vi "Util_Trajectory_WriteFile_Pathweaver.vi"(6 "Trajectory Is Relative":bool, 8 "UtilityWayPoints":T6[](array[typedef]) {"ANGLE" format="%13.3f"; "Y" format="%13.3f"; "X" format="%13.3f"}, 9 "TRAJECTORY":T1 {"States"."POSE"."ROTATION"."SIN" format="%13.4f"; "States"."POSE"."ROTATION"."COS" format="%13.4f"; "States"."POSE"."ROTATION"."VALUE" format="%13.4f"; "States"."POSE"."TRANSLATION"."Y" format="%14.3f"; "States"."POSE"."TRANSLATION"."X" format="%14.3f"; "TotalTImeSecs" format="%20.3f"}, 10 "Comment":string, 11 "Trajectory File Name":path) -> (0 "error out":errorcluster)   [LabVIEW 2019, in "Trajectory_Library.lvlib"]
doc: "Create a CSV file from a Trajectory data structure. This is a special version for Pathweaver created trajectories. This can be used on a PC or the RoboRIO.\n\nParameters:\n - Trajectory - Data structure containing trajectory\n - Trajectory File Name - File name to write to. Existing files are overwritten.\n - Comment - Comment string to include in file comments.\n - Waypoints - waypoints to include in file comments (future)\n - TrajectoryIsRelative - Relative if TRUE otherwise absolute.\n\nReturns:\n - Error out - returned error cluster"
uses:
  Trajectory_Library.lvlib
  DISPLAY_WEIGHTED_WAYPOINT.ctl
  TRANSLATION2D.ctl
  DISPLAY_WAYPOINT.ctl
  ROTATION2D.ctl
  POSE2D.ctl
  TRAJ_STATE.ctl
  TRAJECTORY.ctl
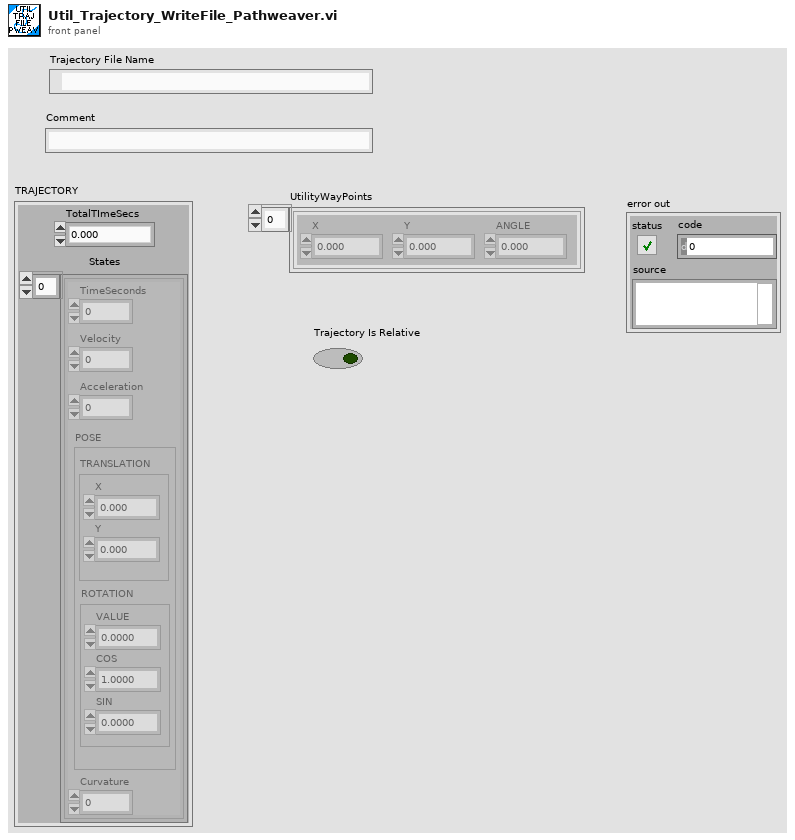
[diagram p1: front panel]
types:
  T1 = typedef "Trajectory_Library.lvlib/TRAJECTORY.ctl" = cluster{"TotalTImeSecs":dbl, "States":T2[]}
  T2 = typedef "Trajectory_Library.lvlib/TRAJ_STATE.ctl" = cluster{"TimeSeconds":dbl, "Velocity":dbl, "Acceleration":dbl, "POSE":T3, "Curvature":dbl}
  T3 = typedef "Trajectory_Library.lvlib/POSE2D.ctl" = cluster{"TRANSLATION":T4, "ROTATION":T5}
  T4 = typedef "Trajectory_Library.lvlib/TRANSLATION2D.ctl" = cluster{"X":dbl, "Y":dbl}
  T5 = typedef "Trajectory_Library.lvlib/ROTATION2D.ctl" = cluster{"VALUE":dbl, "COS":dbl, "SIN":dbl}
  T6 = typedef "Trajectory_Library.lvlib/DISPLAY_WAYPOINT.ctl" = cluster{"X":dbl, "Y":dbl, "ANGLE":dbl}
  T7 = enum16{"open", "replace", "create", "open or create", "replace or create", "replace or create with confirmation"}
  T8 = typedef "Trajectory_Library.lvlib/DISPLAY_WEIGHTED_WAYPOINT.ctl" = cluster{"X":dbl, "Y":dbl, "ANGLE":dbl, "WEIGHT":dbl}
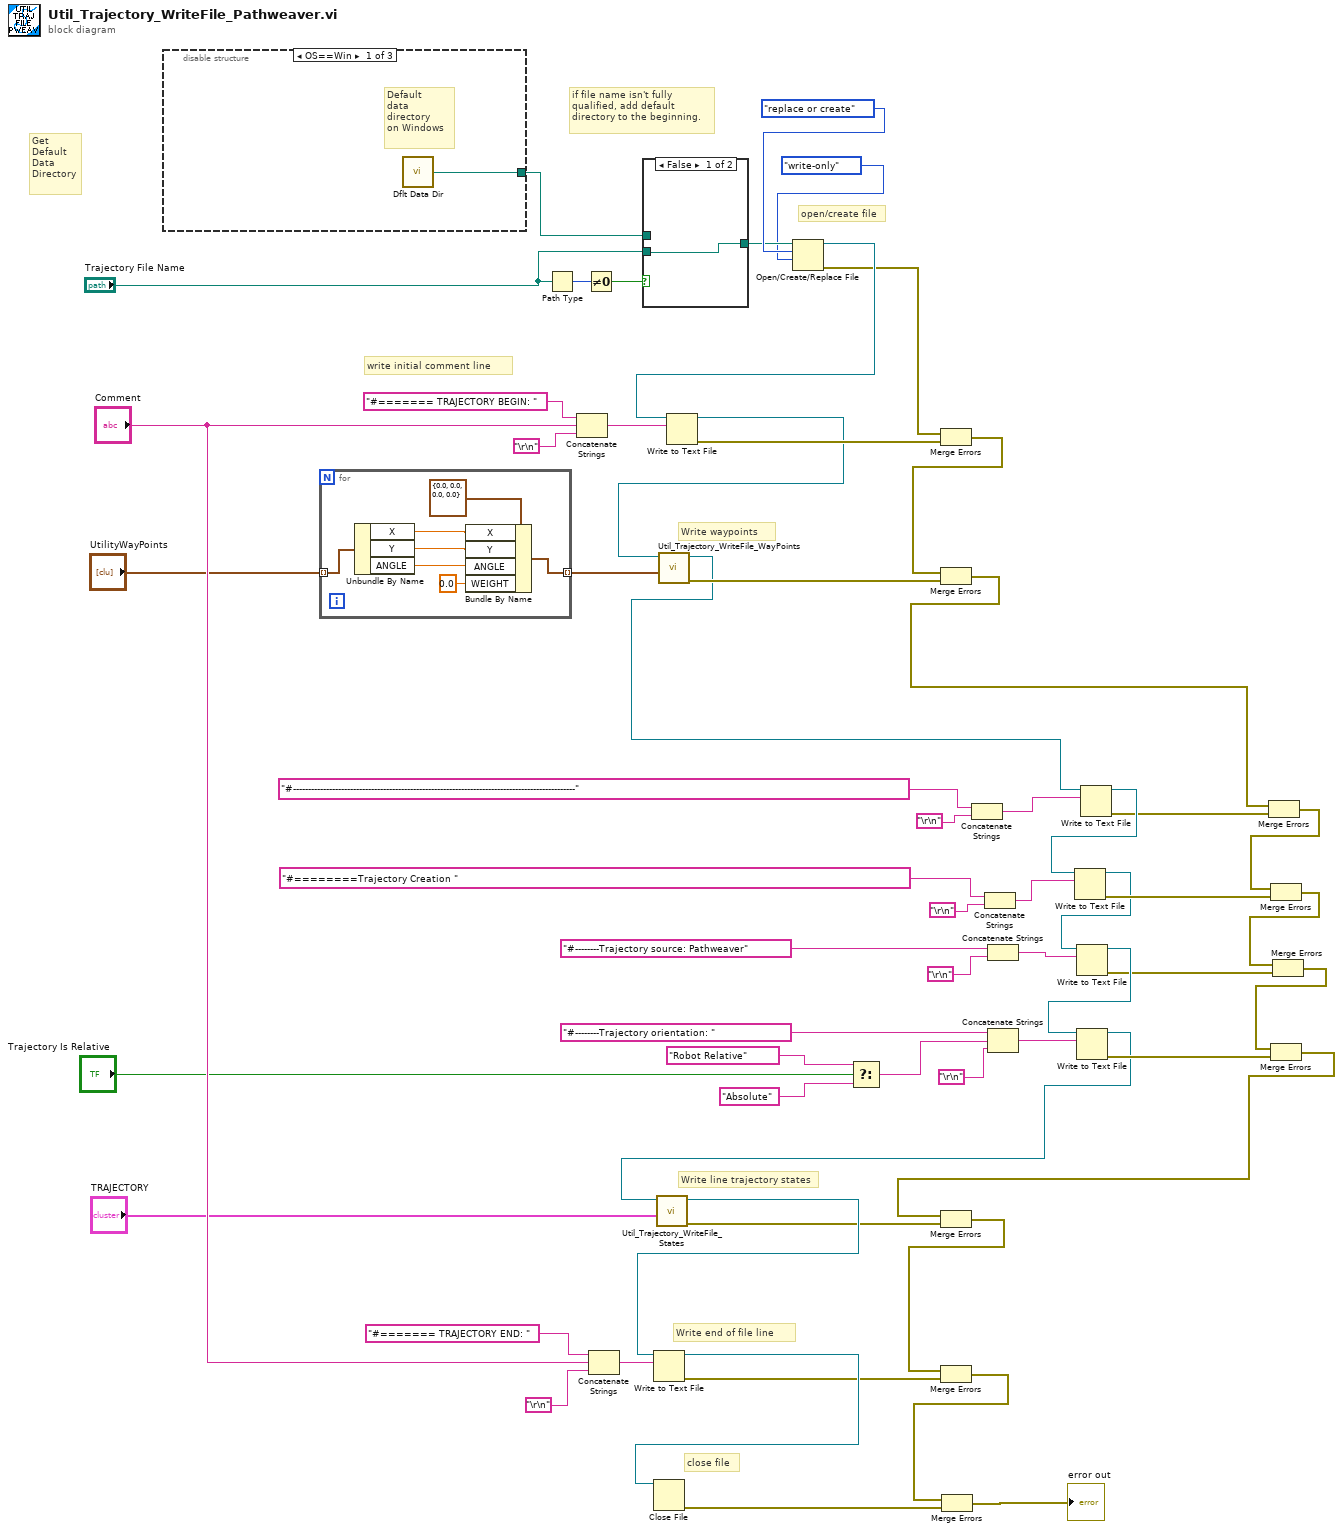
[diagram p0: block diagram]
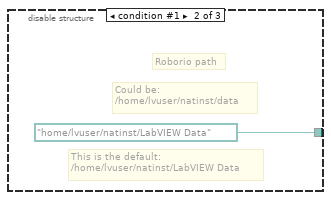
[diagram p2: hidden frame]
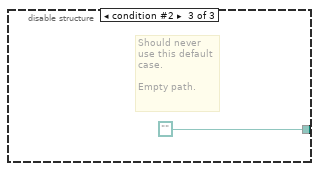
[diagram p3: hidden frame]
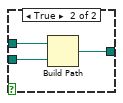
[diagram p4: hidden frame]
diagram:
  # "Write line trajectory states"
  # "open/create file"
  # "if file name isn't fully \nqualified, add default\ndirectory to the beginning."
  # "Get\nDefault\nData\nDirectory"
  # "Write waypoints"
  # "close file"
  # "Write end of file line"
  # "write initial comment line"
  n1 = disable-structure shown="OS==Win" {
    disable-tunnel: [w62 path "/home/lvuser/natinst/LabVIEW Data" path ""] -> w51
    frame condition #0 (active) {
      # "Default\ndata\ndirectory\non Windows"
      n2 = call <vilib>:"Dflt Data Dir.vi"() -> ("App:Default Data Directory"=w62:path)
    }
    frame condition #1 {
      # "This is the default:\n/home/lvuser/natinst/LabVIEW Data"
      # "Could be:\n/home/lvuser/natinst/data"
      # "Roborio path"
    }
    frame condition #2 {
      # "Should never\nuse this default\ncase.\n\nEmpty path."
    }
  }
  n3 = for {
    tunnel: "UtilityWayPoints" -> [w70] mode=indexing
    tunnel: [w65] -> w2 mode=indexing
    n4 = Unbundle By Name(w70) -> ("X"=w69:dbl, "Y"=w68:dbl, "ANGLE"=w67:dbl)
    n5 = Bundle By Name(cluster=T8 {"X"=0.0, "Y"=0.0, "ANGLE"=0.0, "WEIGHT"=0.0} ("UTIL_WEIGHTED_WAYPOINT"), "X"=w69, "Y"=w68, "ANGLE"=w67, "WEIGHT"=0.0) -> (w65:T8)
  }
  n6 = Path Type(1:"Trajectory File Name") -> (0:w54:i16)
  n7 = Concatenate Strings("#======= TRAJECTORY BEGIN: " ("string"), "Comment", "\r\n") -> (w59:string)
  n8 = Not Equal To 0?(x=w54) -> (x != 0?=w53:bool)
  n9 = Concatenate Strings("#======= TRAJECTORY END: " ("string"), "Comment", "\r\n") -> (w55:string)
  n10 = case shown="False" w53 {
    tunnel: [w72 w75] -> w50
    tunnel: w51 -> [_ w74]
    tunnel: "Trajectory File Name" -> [w72 w73]
    frame False {
    }
    frame True {
      n11 = Build Path(base path=w74, name or relative path=w73) -> (appended path=w75:path)
    }
  }
  n12 = Open/Create/Replace File(file path (use dialog)=w50, operation (0:open)=T7."replace or create", access (0:read/write)=enum16{"read/write", "read-only", "write-only"}."write-only") -> (refnum out=w48:refnum<file>, error out=w43:errorcluster)  [unwired: 3 in, 1 out]
  n13 = Write to Text File(file (use dialog)=w48, text=w59) -> (refnum out=w34:refnum<file>, error out=w44:errorcluster)  [unwired: 2 in, 1 out]
  n14 = call "Util_Trajectory_WriteFile_WayPoints.vi"("UtilityWayPoints"=w2, "Byte Steam File In"=w34) -> ("error out"=w42:errorcluster, "Byte Steam File Out"=w4:refnum<file>)  [unwired: 8 in]
  n15 = Select(t="Robot Relative" ("string"), s="Trajectory Is Relative", f="Absolute" ("string")) -> (s? t:f=w24:string)
  n16 = Merge Errors(w43, w44) -> (w35:errorcluster)
  n17 = Merge Errors(w35, w42) -> (w3:errorcluster)
  n18 = Concatenate Strings("#----------------------------------------------------------------------------------------------" ("string"), "\r\n") -> (w28:string)
  n19 = Concatenate Strings("#========Trajectory Creation " ("string"), "\r\n") -> (w31:string)
  n20 = Concatenate Strings("#--------Trajectory source: Pathweaver" ("string"), "\r\n") -> (w13:string)
  n21 = Concatenate Strings("#--------Trajectory orientation: " ("string"), w24, "\r\n") -> (w26:string)
  n22 = Write to Text File(file (use dialog)=w4, text=w28) -> (refnum out=w20:refnum<file>, error out=w18:errorcluster)  [unwired: 2 in, 1 out]
  n23 = Write to Text File(file (use dialog)=w20, text=w31) -> (refnum out=w10:refnum<file>, error out=w19:errorcluster)  [unwired: 2 in, 1 out]
  n24 = Write to Text File(file (use dialog)=w10, text=w13) -> (refnum out=w9:refnum<file>, error out=w8:errorcluster)  [unwired: 2 in, 1 out]
  n25 = Write to Text File(file (use dialog)=w9, text=w26) -> (refnum out=w16:refnum<file>, error out=w25:errorcluster)  [unwired: 2 in, 1 out]
  n26 = call "Util_Trajectory_WriteFile_States.vi"("Trajectory"="TRAJECTORY", "Byte Steam File In"=w16) -> ("error out"=w41:errorcluster, "Byte Steam File Out"=w46:refnum<file>)  [unwired: 8 in]
  n27 = Write to Text File(file (use dialog)=w46, text=w55) -> (refnum out=w45:refnum<file>, error out=w39:errorcluster)  [unwired: 2 in, 1 out]
  n28 = Close File(refnum=w45) -> (error out=w38:errorcluster)  [unwired: 1 in, 1 out]
  n29 = Merge Errors(w3, w18) -> (w17:errorcluster)
  n30 = Merge Errors(w17, w19) -> (w7:errorcluster)
  n31 = Merge Errors(w7, w8) -> (w6:errorcluster)
  n32 = Merge Errors(w6, w25) -> (w14:errorcluster)
  n33 = Merge Errors(w14, w41) -> (w40:errorcluster)
  n34 = Merge Errors(w40, w39) -> (w37:errorcluster)
  n35 = Merge Errors(w37, w38) -> (→"error out":errorcluster)
